vi "20220815-335-read and save temppoint.vi"() -> ()   [LabVIEW 2019]
panel:
  out "Numeric":i32
  out "before substring":string
  out "read buffer 2":string
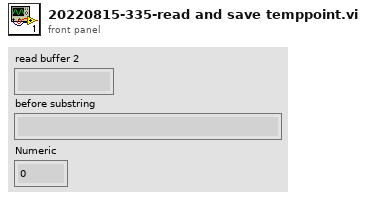
[diagram p1: front panel]
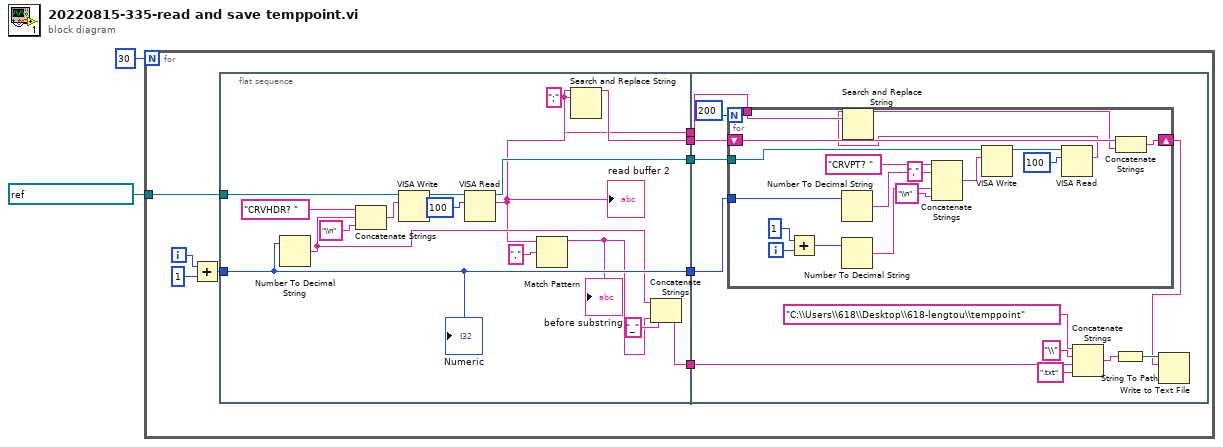
[diagram p0: block diagram]
diagram:
  n1 = for {
    N: 30 -> [_]
    tunnel: refnum<visa-resource-name> "GPIB1::12::INSTR" ("VISA resource name") -> [w11]
    i -> [w10]
    n2 = Add(x=w10, y=1) -> (x+y=w8:i32)
    n3 = flat-sequence {
      tunnel: w8 -> [w25]
      tunnel: w11 -> [w20]
      tunnel: [w25] -> w7
      tunnel: [w21] -> w6
      tunnel: [w15] -> w5
      tunnel: [w13] -> w4
      tunnel: [w12] -> w3
      tunnel: w7 -> [w38]
      tunnel: w6 -> [w39]
      tunnel: w5 -> [w35]
      tunnel: w4 -> [w32]
      tunnel: w3 -> [w28]
      frame #0 {
        w12 = ";" ("search string")
        n4 = Number To Decimal String(number=w25) -> (decimal integer string=w18:string)  [unwired: 1 in]
        n5 = Concatenate Strings("CRVHDR? " ("write buffer"), w18, "\\n" ("string")) -> (w24:string)
        n6 = VISA Write(VISA resource name=w20, write buffer=w24) -> (VISA resource name out=w23:refnum<visa-resource-name>)  [unwired: 1 in, 2 out]
        n7 = VISA Read(VISA resource name=w23, byte count=u32 100) -> (VISA resource name out=w21:refnum<visa-resource-name>, read buffer=w14:string)  [unwired: 1 in, 2 out]
        "read buffer 2" <- w14
        n8 = Match Pattern(string=w14, regular expression=",") -> (before substring=w16:string)  [unwired: 1 in, 3 out]
        "before substring" <- w16
        n9 = Search and Replace String(input string=w14, search string=w12) -> (result string=w13:string)  [unwired: 6 in, 3 out]
        n10 = Concatenate Strings(w18, "_" ("string"), w16) -> (w15:string)
        "Numeric" <- w25
      }
      frame #1 {
        n11 = for {
          N: 200 -> [_]
          tunnel: w39 -> [w57]
          tunnel: w38 -> [w52]
          shift-right: [w44] -> w31
          shift-left: w32 -> [w45]
          tunnel: w28 -> [w42]
          i -> [w54]
          n12 = Add(x=1, y=w54) -> (x+y=w50:i32)
          n13 = Number To Decimal String(number=w52) -> (decimal integer string=w51:string)  [unwired: 1 in]
          n14 = Number To Decimal String(number=w50) -> (decimal integer string=w49:string)  [unwired: 1 in]
          n15 = Concatenate Strings("CRVPT? " ("write buffer"), w51, "," ("string"), w49, "\\n" ("string")) -> (w46:string)
          n16 = VISA Write(VISA resource name=w57, write buffer=w46) -> (VISA resource name out=w56:refnum<visa-resource-name>)  [unwired: 1 in, 2 out]
          n17 = VISA Read(VISA resource name=w56, byte count=u32 100) -> (read buffer=w41:string)  [unwired: 1 in, 3 out]
          n18 = Search and Replace String(input string=w41, search string=w42) -> (result string=w40:string)  [unwired: 6 in, 3 out]
          n19 = Concatenate Strings(w45, w40) -> (w44:string)
        }
        n20 = Concatenate Strings("C:\\Users\\618\\Desktop\\618-lengtou\\temppoint" ("string"), "\\" ("string"), w35, ".txt" ("string")) -> (w34:string)
        n21 = String To Path(string=w34) -> (path=w33:path)
        n22 = Write to Text File(file (use dialog)=w33, text=w31) -> ()  [unwired: 2 in, 3 out]
      }
    }
  }
